vi "fgv_waypoint_total.vi"(7 "cmd":enum16{"write", "read"}(ring), 11 "waypoint total in":cluster{"waypt":cluster{"X":dbl, "Y":dbl}[]}[](array[cluster])) -> (3 "waypoint total out":cluster{"waypt":cluster{"X":dbl, "Y":dbl}[]}[](array[cluster]))   [LabVIEW 2019]
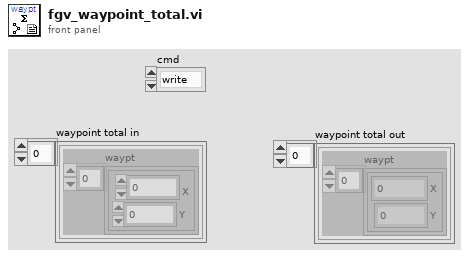
[diagram p1: front panel]
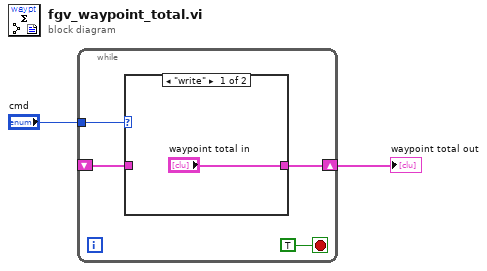
[diagram p0: block diagram]
diagram:
  n1 = while {
    tunnel: "cmd" -> [w5]
    shift-right: [w4] -> w1
    shift-left: _ -> [w3]
    stop <- TRUE stop-if-true
    n2 = case shown="\"write\"" w5 {
      tunnel: ["waypoint total in" w8] -> w4
      tunnel: w3 -> [_ w8]
      frame "write" {
      }
      frame "read", Default {
      }
    }
  }
  "waypoint total out" <- w1
